vi "Update Data File to add Financials.vi"() -> ()   [LabVIEW 2020]
uses:
  WPC Player and Financial Stats.ctl
panel:
  in  "file path (use dialog)":path=path "G:/My Drive/WPC Stat Scrape/Data/WPC Stats.bin"
  out "error out":errorcluster
  out "WPC Player and Financial Stats":T1[][](array[typedef])=[[{"Player Name"="Andrew", "Date Updated"=timestamp(3695932800 s since 1904-01-01), "Tournament Stats"={"Hands Won"=674, "Hands Played"=2024, "Hands Dealt"=5109, "All-Ins"=149, "Entered"=36, "Winnings"=785.66, "Profit"=-679.15}, "Cash Stats"={"Hands Won"=1363, "Hands Played"=4015, "Hands Dealt"=9376, "All-Ins"=232, "Profit"=-195.0}}, {"Player Name"="Brian", "Date Updated"=timestamp(3695932800 s since 1904-01-01), "Tournament Stats"={"Hands Won"=936, "Hands Played"=2541, "Hands Dealt"=5628, "All-Ins"=306, "Entered"=47, "Winnings"=1307.11, "Profit"=-47.7}, "Cash Stats"={"Hands Won"=2327, "Hands Played"=6457, "Hands Dealt"=11257, "All-Ins"=405, "Profit"=1902.25}}, {"Player Name"="Daniel", "Date Updated"=timestamp(3695932800 s since 1904-01-01), "Tournament Stats"={"Hands Won"=94, "Hands Played"=308, "Hands Dealt"=723, "All-Ins"=23, "Entered"=6, "Winnings"=320.0, "Profit"=-20.0}, "Cash Stats"={"Hands Won"=0, "Hands Played"=0, "Hands Dealt"=0, "All-Ins"=0, "Profit"=0.0}}, {"Player Name"="David", "Date Updated"=timestamp(3695932800 s since 1904-01-01), "Tournament Stats"={"Hands Won"=898, "Hands Played"=2002, "Hands Dealt"=4936, "All-Ins"=188, "Entered"=37, "Winnings"=1934.16, "Profit"=574.16}, "Cash Stats"={"Hands Won"=0, "Hands Played"=0, "Hands Dealt"=0, "All-Ins"=0, "Profit"=0.0}}, {"Player Name"="Dennis", "Date Updated"=timestamp(3695932800 s since 1904-01-01), "Tournament Stats"={"Hands Won"=266, "Hands Played"=670, "Hands Dealt"=1843, "All-Ins"=55, "Entered"=13, "Winnings"=1351.83, "Profit"=617.02}, "Cash Stats"={"Hands Won"=34, "Hands Played"=114, "Hands Dealt"=216, "All-Ins"=11, "Profit"=-12.75}}, {"Player Name"="Doug", "Date Updated"=timestamp(3695932800 s since 1904-01-01), "Tournament Stats"={"Hands Won"=144, "Hands Played"=441, "Hands Dealt"=722, "All-Ins"=44, "Entered"=11, "Winnings"=225.0, "Profit"=-89.81}, "Cash Stats"={"Hands Won"=120, "Hands Played"=285, "Hands Dealt"=428, "All-Ins"=22, "Profit"=-39.5}}, {"Player Name"="Erik", "Date Updated"=timestamp(3695932800 s since 1904-01-01), "Tournament Stats"={"Hands Won"=180, "Hands Played"=626, "Hands Dealt"=1825, "All-Ins"=72, "Entered"=14, "Winnings"=200.66, "Profit"=-259.34}, "Cash Stats"={"Hands Won"=11, "Hands Played"=43, "Hands Dealt"=98, "All-Ins"=7, "Profit"=-34.75}}, {"Player Name"="Ethan", "Date Updated"=timestamp(3695932800 s since 1904-01-01), "Tournament Stats"={"Hands Won"=735, "Hands Played"=2022, "Hands Dealt"=5107, "All-Ins"=210, "Entered"=41, "Winnings"=1270.72, "Profit"=195.91}, "Cash Stats"={"Hands Won"=2067, "Hands Played"=5488, "Hands Dealt"=10831, "All-Ins"=624, "Profit"=1356.0}}, {"Player Name"="Ian", "Date Updated"=timestamp(3695932800 s since 1904-01-01), "Tournament Stats"={"Hands Won"=1572, "Hands Played"=4650, "Hands Dealt"=8870, "All-Ins"=332, "Entered"=69, "Winnings"=1957.52, "Profit"=-407.29}, "Cash Stats"={"Hands Won"=129, "Hands Played"=435, "Hands Dealt"=646, "All-Ins"=23, "Profit"=-112.0}}, {"Player Name"="Ira", "Date Updated"=timestamp(3695932800 s since 1904-01-01), "Tournament Stats"={"Hands Won"=1430, "Hands Played"=3509, "Hands Dealt"=8784, "All-Ins"=341, "Entered"=72, "Winnings"=2796.14, "Profit"=491.33}, "Cash Stats"={"Hands Won"=1, "Hands Played"=3, "Hands Dealt"=6, "All-Ins"=1, "Profit"=-20.0}}, {"Player Name"="Jason", "Date Updated"=timestamp(3695932800 s since 1904-01-01), "Tournament Stats"={"Hands Won"=137, "Hands Played"=440, "Hands Dealt"=846, "All-Ins"=37, "Entered"=10, "Winnings"=56.0, "Profit"=-324.0}, "Cash Stats"={"Hands Won"=87, "Hands Played"=305, "Hands Dealt"=448, "All-Ins"=19, "Profit"=-77.75}}, {"Player Name"="Jeff", "Date Updated"=timestamp(3695932800 s since 1904-01-01), "Tournament Stats"={"Hands Won"=445, "Hands Played"=1629, "Hands Dealt"=3147, "All-Ins"=145, "Entered"=39, "Winnings"=420.0, "Profit"=-584.81}, "Cash Stats"={"Hands Won"=0, "Hands Played"=0, "Hands Dealt"=0, "All-Ins"=0, "Profit"=0.0}}, {"Player Name"="Jeff-R", "Date Updated"=timestamp(3695932800 s since 1904-01-01), "Tournament Stats"={"Hands Won"=134, "Hands Played"=331, "Hands Dealt"=875, "All-Ins"=43, "Entered"=7, "Winnings"=256.66, "Profit"=-3.34}, "Cash Stats"={"Hands Won"=10, "Hands Played"=25, "Hands Dealt"=60, "All-Ins"=3, "Profit"=-40.0}}, {"Player Name"="Joe", "Date Updated"=timestamp(3695932800 s since 1904-01-01), "Tournament Stats"={"Hands Won"=7, "Hands Played"=25, "Hands Dealt"=96, "All-Ins"=4, "Entered"=1, "Winnings"=0.0, "Profit"=-60.0}, "Cash Stats"={"Hands Won"=40, "Hands Played"=136, "Hands Dealt"=192, "All-Ins"=13, "Profit"=-132.5}}, {"Player Name"="Joe-Hockman", "Date Updated"=timestamp(3695932800 s since 1904-01-01), "Tournament Stats"={"Hands Won"=0, "Hands Played"=0, "Hands Dealt"=0, "All-Ins"=0, "Entered"=0, "Winnings"=0.0, "Profit"=-40.0}, "Cash Stats"={"Hands Won"=0, "Hands Played"=0, "Hands Dealt"=0, "All-Ins"=0, "Profit"=0.0}}, {"Player Name"="Jonathan-H", "Date Updated"=timestamp(3695932800 s since 1904-01-01), "Tournament Stats"={"Hands Won"=1295, "Hands Played"=2760, "Hands Dealt"=8906, "All-Ins"=385, "Entered"=70, "Winnings"=3077.49, "Profit"=762.68}, "Cash Stats"={"Hands Won"=2243, "Hands Played"=5750, "Hands Dealt"=9974, "All-Ins"=451, "Profit"=1226.5}}, {"Player Name"="Jonathan-M", "Date Updated"=timestamp(3695932800 s since 1904-01-01), "Tournament Stats"={"Hands Won"=2012, "Hands Played"=4111, "Hands Dealt"=8961, "All-Ins"=623, "Entered"=72, "Winnings"=3723.66, "Profit"=1128.85}, "Cash Stats"={"Hands Won"=5567, "Hands Played"=10633, "Hands Dealt"=14708, "All-Ins"=1306, "Profit"=-4255.25}}, {"Player Name"="Mark", "Date Updated"=timestamp(3695932800 s since 1904-01-01), "Tournament Stats"={"Hands Won"=1072, "Hands Played"=2139, "Hands Dealt"=6063, "All-Ins"=291, "Entered"=43, "Winnings"=3075.83, "Profit"=1615.83}, "Cash Stats"={"Hands Won"=746, "Hands Played"=1778, "Hands Dealt"=3876, "All-Ins"=94, "Profit"=895.25}}, {"Player Name"="Marty", "Date Updated"=timestamp(3695932800 s since 1904-01-01), "Tournament Stats"={"Hands Won"=1333, "Hands Played"=3356, "Hands Dealt"=8693, "All-Ins"=359, "Entered"=63, "Winnings"=2027.99, "Profit"=197.99}, "Cash Stats"={"Hands Won"=177, "Hands Played"=535, "Hands Dealt"=1236, "All-Ins"=35, "Profit"=-120.25}}, {"Player Name"="Matt-H", "Date Updated"=timestamp(3695932800 s since 1904-01-01), "Tournament Stats"={"Hands Won"=54, "Hands Played"=147, "Hands Dealt"=285, "All-Ins"=9, "Entered"=4, "Winnings"=34.0, "Profit"=-66.0}, "Cash Stats"={"Hands Won"=0, "Hands Played"=0, "Hands Dealt"=0, "All-Ins"=0, "Profit"=0.0}}, {"Player Name"="Matt-R", "Date Updated"=timestamp(3695932800 s since 1904-01-01), "Tournament Stats"={"Hands Won"=1041, "Hands Played"=2491, "Hands Dealt"=7307, "All-Ins"=340, "Entered"=50, "Winnings"=1520.16, "Profit"=-274.65}, "Cash Stats"={"Hands Won"=264, "Hands Played"=640, "Hands Dealt"=1515, "All-Ins"=91, "Profit"=-121.0}}, {"Player Name"="MikeDolan", "Date Updated"=timestamp(3695932800 s since 1904-01-01), "Tournament Stats"={"Hands Won"=529, "Hands Played"=1505, "Hands Dealt"=3790, "All-Ins"=171, "Entered"=26, "Winnings"=1025.66, "Profit"=85.66}, "Cash Stats"={"Hands Won"=32, "Hands Played"=117, "Hands Dealt"=225, "All-Ins"=14, "Profit"=-66.0}}, {"Player Name"="Nate", "Date Updated"=timestamp(3695932800 s since 1904-01-01), "Tournament Stats"={"Hands Won"=184, "Hands Played"=494, "Hands Dealt"=1384, "All-Ins"=42, "Entered"=14, "Winnings"=234.0, "Profit"=-36.0}, "Cash Stats"={"Hands Won"=0, "Hands Played"=0, "Hands Dealt"=0, "All-Ins"=0, "Profit"=0.0}}, {"Player Name"="Oren", "Date Updated"=timestamp(3695932800 s since 1904-01-01), "Tournament Stats"={"Hands Won"=822, "Hands Played"=1902, "Hands Dealt"=5455, "All-Ins"=177, "Entered"=46, "Winnings"=1157.32, "Profit"=-497.49}, "Cash Stats"={"Hands Won"=19, "Hands Played"=76, "Hands Dealt"=168, "All-Ins"=10, "Profit"=-140.0}}, {"Player Name"="Tom", "Date Updated"=timestamp(3695932800 s since 1904-01-01), "Tournament Stats"={"Hands Won"=0, "Hands Played"=0, "Hands Dealt"=0, "All-Ins"=0, "Entered"=0, "Winnings"=0.0, "Profit"=-120.0}, "Cash Stats"={"Hands Won"=0, "Hands Played"=0, "Hands Dealt"=0, "All-Ins"=0, "Profit"=6.75}}], [{"Player Name"="Andrew", "Date Updated"=timestamp(3696278400 s since 1904-01-01), "Tournament Stats"={"Hands Won"=692, "Hands Played"=2072, "Hands Dealt"=5257, "All-Ins"=152, "Entered"=37, "Winnings"=785.66, "Profit"=-679.15}, "Cash Stats"={"Hands Won"=1438, "Hands Played"=4236, "Hands Dealt"=9848, "All-Ins"=241, "Profit"=-195.0}}, {"Player Name"="Brian", "Date Updated"=timestamp(3696278400 s since 1904-01-01), "Tournament Stats"={"Hands Won"=982, "Hands Played"=2638, "Hands Dealt"=5878, "All-Ins"=313, "Entered"=49, "Winnings"=1307.11, "Profit"=-47.7}, "Cash Stats"={"Hands Won"=2444, "Hands Played"=6799, "Hands Dealt"=11839, "All-Ins"=418, "Profit"=1902.25}}, {"Player Name"="Daniel", "Date Updated"=timestamp(3696278400 s since 1904-01-01), "Tournament Stats"={"Hands Won"=123, "Hands Played"=372, "Hands Dealt"=887, "All-Ins"=30, "Entered"=7, "Winnings"=320.0, "Profit"=-20.0}, "Cash Stats"={"Hands Won"=0, "Hands Played"=0, "Hands Dealt"=0, "All-Ins"=0, "Profit"=0.0}}, {"Player Name"="David", "Date Updated"=timestamp(3696278400 s since 1904-01-01), "Tournament Stats"={"Hands Won"=923, "Hands Played"=2058, "Hands Dealt"=5088, "All-Ins"=191, "Entered"=38, "Winnings"=1934.16, "Profit"=574.16}, "Cash Stats"={"Hands Won"=0, "Hands Played"=0, "Hands Dealt"=0, "All-Ins"=0, "Profit"=0.0}}, {"Player Name"="Dennis", "Date Updated"=timestamp(3696278400 s since 1904-01-01), "Tournament Stats"={"Hands Won"=291, "Hands Played"=736, "Hands Dealt"=2087, "All-Ins"=67, "Entered"=15, "Winnings"=1351.83, "Profit"=617.02}, "Cash Stats"={"Hands Won"=64, "Hands Played"=197, "Hands Dealt"=380, "All-Ins"=17, "Profit"=-12.75}}, {"Player Name"="Doug", "Date Updated"=timestamp(3696278400 s since 1904-01-01), "Tournament Stats"={"Hands Won"=144, "Hands Played"=441, "Hands Dealt"=722, "All-Ins"=44, "Entered"=11, "Winnings"=225.0, "Profit"=-89.81}, "Cash Stats"={"Hands Won"=120, "Hands Played"=285, "Hands Dealt"=428, "All-Ins"=22, "Profit"=-39.5}}, {"Player Name"="Erik", "Date Updated"=timestamp(3696278400 s since 1904-01-01), "Tournament Stats"={"Hands Won"=187, "Hands Played"=660, "Hands Dealt"=1934, "All-Ins"=74, "Entered"=15, "Winnings"=200.66, "Profit"=-259.34}, "Cash Stats"={"Hands Won"=11, "Hands Played"=43, "Hands Dealt"=98, "All-Ins"=7, "Profit"=-34.75}}, {"Player Name"="Ethan", "Date Updated"=timestamp(3696278400 s since 1904-01-01), "Tournament Stats"={"Hands Won"=781, "Hands Played"=2112, "Hands Dealt"=5289, "All-Ins"=214, "Entered"=42, "Winnings"=1270.72, "Profit"=195.91}, "Cash Stats"={"Hands Won"=2170, "Hands Played"=5765, "Hands Dealt"=11302, "All-Ins"=648, "Profit"=1356.0}}, {"Player Name"="Ian", "Date Updated"=timestamp(3696278400 s since 1904-01-01), "Tournament Stats"={"Hands Won"=1605, "Hands Played"=4769, "Hands Dealt"=9117, "All-Ins"=349, "Entered"=71, "Winnings"=1957.52, "Profit"=-407.29}, "Cash Stats"={"Hands Won"=131, "Hands Played"=450, "Hands Dealt"=675, "All-Ins"=24, "Profit"=-112.0}}, {"Player Name"="Ira", "Date Updated"=timestamp(3696278400 s since 1904-01-01), "Tournament Stats"={"Hands Won"=1453, "Hands Played"=3592, "Hands Dealt"=8981, "All-Ins"=350, "Entered"=74, "Winnings"=2796.14, "Profit"=491.33}, "Cash Stats"={"Hands Won"=1, "Hands Played"=3, "Hands Dealt"=6, "All-Ins"=1, "Profit"=-20.0}}, {"Player Name"="Jason", "Date Updated"=timestamp(3696278400 s since 1904-01-01), "Tournament Stats"={"Hands Won"=137, "Hands Played"=440, "Hands Dealt"=846, "All-Ins"=37, "Entered"=10, "Winnings"=56.0, "Profit"=-324.0}, "Cash Stats"={"Hands Won"=87, "Hands Played"=305, "Hands Dealt"=448, "All-Ins"=19, "Profit"=-77.75}}, {"Player Name"="Jeff", "Date Updated"=timestamp(3696278400 s since 1904-01-01), "Tournament Stats"={"Hands Won"=460, "Hands Played"=1685, "Hands Dealt"=3258, "All-Ins"=150, "Entered"=40, "Winnings"=420.0, "Profit"=-584.81}, "Cash Stats"={"Hands Won"=0, "Hands Played"=0, "Hands Dealt"=0, "All-Ins"=0, "Profit"=0.0}}, {"Player Name"="Jeff-R", "Date Updated"=timestamp(3696278400 s since 1904-01-01), "Tournament Stats"={"Hands Won"=134, "Hands Played"=331, "Hands Dealt"=875, "All-Ins"=43, "Entered"=7, "Winnings"=256.66, "Profit"=-3.34}, "Cash Stats"={"Hands Won"=10, "Hands Played"=25, "Hands Dealt"=60, "All-Ins"=3, "Profit"=-40.0}}, {"Player Name"="Joe", "Date Updated"=timestamp(3696278400 s since 1904-01-01), "Tournament Stats"={"Hands Won"=7, "Hands Played"=25, "Hands Dealt"=96, "All-Ins"=4, "Entered"=1, "Winnings"=0.0, "Profit"=-60.0}, "Cash Stats"={"Hands Won"=40, "Hands Played"=136, "Hands Dealt"=192, "All-Ins"=13, "Profit"=-132.5}}, {"Player Name"="Joe-Hockman", "Date Updated"=timestamp(3696278400 s since 1904-01-01), "Tournament Stats"={"Hands Won"=0, "Hands Played"=0, "Hands Dealt"=0, "All-Ins"=0, "Entered"=0, "Winnings"=0.0, "Profit"=-40.0}, "Cash Stats"={"Hands Won"=0, "Hands Played"=0, "Hands Dealt"=0, "All-Ins"=0, "Profit"=0.0}}, {"Player Name"="Jonathan-H", "Date Updated"=timestamp(3696278400 s since 1904-01-01), "Tournament Stats"={"Hands Won"=1355, "Hands Played"=2840, "Hands Dealt"=9179, "All-Ins"=393, "Entered"=72, "Winnings"=3077.49, "Profit"=762.68}, "Cash Stats"={"Hands Won"=2263, "Hands Played"=5817, "Hands Dealt"=10092, "All-Ins"=461, "Profit"=1226.5}}, {"Player Name"="Jonathan-M", "Date Updated"=timestamp(3696278400 s since 1904-01-01), "Tournament Stats"={"Hands Won"=2058, "Hands Played"=4217, "Hands Dealt"=9164, "All-Ins"=642, "Entered"=74, "Winnings"=3723.66, "Profit"=1128.85}, "Cash Stats"={"Hands Won"=5684, "Hands Played"=10939, "Hands Dealt"=15071, "All-Ins"=1333, "Profit"=-4255.25}}, {"Player Name"="Mark", "Date Updated"=timestamp(3696278400 s since 1904-01-01), "Tournament Stats"={"Hands Won"=1081, "Hands Played"=2168, "Hands Dealt"=6180, "All-Ins"=297, "Entered"=44, "Winnings"=3075.83, "Profit"=1615.83}, "Cash Stats"={"Hands Won"=836, "Hands Played"=1984, "Hands Dealt"=4426, "All-Ins"=100, "Profit"=895.25}}, {"Player Name"="Marty", "Date Updated"=timestamp(3696278400 s since 1904-01-01), "Tournament Stats"={"Hands Won"=1391, "Hands Played"=3485, "Hands Dealt"=9040, "All-Ins"=374, "Entered"=65, "Winnings"=2027.99, "Profit"=197.99}, "Cash Stats"={"Hands Won"=189, "Hands Played"=570, "Hands Dealt"=1351, "All-Ins"=38, "Profit"=-120.25}}, {"Player Name"="Matt-H", "Date Updated"=timestamp(3696278400 s since 1904-01-01), "Tournament Stats"={"Hands Won"=54, "Hands Played"=147, "Hands Dealt"=285, "All-Ins"=9, "Entered"=4, "Winnings"=34.0, "Profit"=-66.0}, "Cash Stats"={"Hands Won"=0, "Hands Played"=0, "Hands Dealt"=0, "All-Ins"=0, "Profit"=0.0}}, {"Player Name"="Matt-R", "Date Updated"=timestamp(3696278400 s since 1904-01-01), "Tournament Stats"={"Hands Won"=1056, "Hands Played"=2563, "Hands Dealt"=7489, "All-Ins"=347, "Entered"=52, "Winnings"=1520.16, "Profit"=-274.65}, "Cash Stats"={"Hands Won"=264, "Hands Played"=640, "Hands Dealt"=1515, "All-Ins"=91, "Profit"=-121.0}}, {"Player Name"="MikeDolan", "Date Updated"=timestamp(3696278400 s since 1904-01-01), "Tournament Stats"={"Hands Won"=555, "Hands Played"=1565, "Hands Dealt"=3960, "All-Ins"=178, "Entered"=27, "Winnings"=1025.66, "Profit"=85.66}, "Cash Stats"={"Hands Won"=32, "Hands Played"=117, "Hands Dealt"=225, "All-Ins"=14, "Profit"=-66.0}}, {"Player Name"="Nate", "Date Updated"=timestamp(3696278400 s since 1904-01-01), "Tournament Stats"={"Hands Won"=184, "Hands Played"=494, "Hands Dealt"=1384, "All-Ins"=42, "Entered"=14, "Winnings"=234.0, "Profit"=-36.0}, "Cash Stats"={"Hands Won"=0, "Hands Played"=0, "Hands Dealt"=0, "All-Ins"=0, "Profit"=0.0}}, {"Player Name"="Oren", "Date Updated"=timestamp(3696278400 s since 1904-01-01), "Tournament Stats"={"Hands Won"=850, "Hands Played"=1972, "Hands Dealt"=5639, "All-Ins"=182, "Entered"=48, "Winnings"=1157.32, "Profit"=-497.49}, "Cash Stats"={"Hands Won"=19, "Hands Played"=76, "Hands Dealt"=168, "All-Ins"=10, "Profit"=-140.0}}, {"Player Name"="Tom", "Date Updated"=timestamp(3696278400 s since 1904-01-01), "Tournament Stats"={"Hands Won"=0, "Hands Played"=0, "Hands Dealt"=0, "All-Ins"=0, "Entered"=0, "Winnings"=0.0, "Profit"=-120.0}, "Cash Stats"={"Hands Won"=0, "Hands Played"=0, "Hands Dealt"=0, "All-Ins"=0, "Profit"=6.75}}], [{"Player Name"="Andrew", "Date Updated"=timestamp(3696883200 s since 1904-01-01), "Tournament Stats"={"Hands Won"=703, "Hands Played"=2106, "Hands Dealt"=5350, "All-Ins"=156, "Entered"=38, "Winnings"=785.66, "Profit"=-679.15}, "Cash Stats"={"Hands Won"=1504, "Hands Played"=4457, "Hands Dealt"=10311, "All-Ins"=259, "Profit"=-195.0}}, {"Player Name"="Brian", "Date Updated"=timestamp(3696883200 s since 1904-01-01), "Tournament Stats"={"Hands Won"=989, "Hands Played"=2670, "Hands Dealt"=5940, "All-Ins"=317, "Entered"=50, "Winnings"=1307.11, "Profit"=-47.7}, "Cash Stats"={"Hands Won"=2519, "Hands Played"=7033, "Hands Dealt"=12257, "All-Ins"=421, "Profit"=1902.25}}, {"Player Name"="Daniel", "Date Updated"=timestamp(3696883200 s since 1904-01-01), "Tournament Stats"={"Hands Won"=123, "Hands Played"=372, "Hands Dealt"=887, "All-Ins"=30, "Entered"=7, "Winnings"=320.0, "Profit"=-20.0}, "Cash Stats"={"Hands Won"=0, "Hands Played"=0, "Hands Dealt"=0, "All-Ins"=0, "Profit"=0.0}}, {"Player Name"="David", "Date Updated"=timestamp(3696883200 s since 1904-01-01), "Tournament Stats"={"Hands Won"=930, "Hands Played"=2085, "Hands Dealt"=5181, "All-Ins"=193, "Entered"=39, "Winnings"=1934.16, "Profit"=574.16}, "Cash Stats"={"Hands Won"=0, "Hands Played"=0, "Hands Dealt"=0, "All-Ins"=0, "Profit"=0.0}}, {"Player Name"="Dennis", "Date Updated"=timestamp(3696883200 s since 1904-01-01), "Tournament Stats"={"Hands Won"=319, "Hands Played"=819, "Hands Dealt"=2303, "All-Ins"=72, "Entered"=17, "Winnings"=1351.83, "Profit"=617.02}, "Cash Stats"={"Hands Won"=70, "Hands Played"=213, "Hands Dealt"=407, "All-Ins"=21, "Profit"=-12.75}}, {"Player Name"="Doug", "Date Updated"=timestamp(3696883200 s since 1904-01-01), "Tournament Stats"={"Hands Won"=157, "Hands Played"=475, "Hands Dealt"=808, "All-Ins"=48, "Entered"=12, "Winnings"=225.0, "Profit"=-89.81}, "Cash Stats"={"Hands Won"=120, "Hands Played"=285, "Hands Dealt"=428, "All-Ins"=22, "Profit"=-39.5}}, {"Player Name"="Erik", "Date Updated"=timestamp(3696883200 s since 1904-01-01), "Tournament Stats"={"Hands Won"=187, "Hands Played"=660, "Hands Dealt"=1934, "All-Ins"=74, "Entered"=15, "Winnings"=200.66, "Profit"=-259.34}, "Cash Stats"={"Hands Won"=11, "Hands Played"=43, "Hands Dealt"=98, "All-Ins"=7, "Profit"=-34.75}}, {"Player Name"="Ethan", "Date Updated"=timestamp(3696883200 s since 1904-01-01), "Tournament Stats"={"Hands Won"=847, "Hands Played"=2260, "Hands Dealt"=5600, "All-Ins"=229, "Entered"=44, "Winnings"=1270.72, "Profit"=195.91}, "Cash Stats"={"Hands Won"=2319, "Hands Played"=6069, "Hands Dealt"=11823, "All-Ins"=660, "Profit"=1356.0}}, {"Player Name"="Ian", "Date Updated"=timestamp(3696883200 s since 1904-01-01), "Tournament Stats"={"Hands Won"=1650, "Hands Played"=4899, "Hands Dealt"=9371, "All-Ins"=357, "Entered"=73, "Winnings"=1957.52, "Profit"=-407.29}, "Cash Stats"={"Hands Won"=177, "Hands Played"=584, "Hands Dealt"=866, "All-Ins"=25, "Profit"=-112.0}}, {"Player Name"="Ira", "Date Updated"=timestamp(3696883200 s since 1904-01-01), "Tournament Stats"={"Hands Won"=1477, "Hands Played"=3674, "Hands Dealt"=9138, "All-Ins"=360, "Entered"=76, "Winnings"=2796.14, "Profit"=491.33}, "Cash Stats"={"Hands Won"=1, "Hands Played"=3, "Hands Dealt"=6, "All-Ins"=1, "Profit"=-20.0}}, {"Player Name"="Jason", "Date Updated"=timestamp(3696883200 s since 1904-01-01), "Tournament Stats"={"Hands Won"=137, "Hands Played"=440, "Hands Dealt"=846, "All-Ins"=37, "Entered"=10, "Winnings"=56.0, "Profit"=-324.0}, "Cash Stats"={"Hands Won"=87, "Hands Played"=305, "Hands Dealt"=448, "All-Ins"=19, "Profit"=-77.75}}, {"Player Name"="Jeff", "Date Updated"=timestamp(3696883200 s since 1904-01-01), "Tournament Stats"={"Hands Won"=477, "Hands Played"=1738, "Hands Dealt"=3360, "All-Ins"=155, "Entered"=42, "Winnings"=420.0, "Profit"=-584.81}, "Cash Stats"={"Hands Won"=0, "Hands Played"=0, "Hands Dealt"=0, "All-Ins"=0, "Profit"=0.0}}, {"Player Name"="Jeff-R", "Date Updated"=timestamp(3696883200 s since 1904-01-01), "Tournament Stats"={"Hands Won"=139, "Hands Played"=345, "Hands Dealt"=913, "All-Ins"=45, "Entered"=8, "Winnings"=256.66, "Profit"=-3.34}, "Cash Stats"={"Hands Won"=10, "Hands Played"=25, "Hands Dealt"=60, "All-Ins"=3, "Profit"=-40.0}}, {"Player Name"="Joe", "Date Updated"=timestamp(3696883200 s since 1904-01-01), "Tournament Stats"={"Hands Won"=7, "Hands Played"=25, "Hands Dealt"=96, "All-Ins"=4, "Entered"=1, "Winnings"=0.0, "Profit"=-60.0}, "Cash Stats"={"Hands Won"=40, "Hands Played"=136, "Hands Dealt"=192, "All-Ins"=13, "Profit"=-132.5}}, {"Player Name"="Joe-Hockman", "Date Updated"=timestamp(3696883200 s since 1904-01-01), "Tournament Stats"={"Hands Won"=0, "Hands Played"=0, "Hands Dealt"=0, "All-Ins"=0, "Entered"=0, "Winnings"=0.0, "Profit"=-40.0}, "Cash Stats"={"Hands Won"=0, "Hands Played"=0, "Hands Dealt"=0, "All-Ins"=0, "Profit"=0.0}}, {"Player Name"="Jonathan-H", "Date Updated"=timestamp(3696883200 s since 1904-01-01), "Tournament Stats"={"Hands Won"=1402, "Hands Played"=2937, "Hands Dealt"=9447, "All-Ins"=402, "Entered"=74, "Winnings"=3077.49, "Profit"=762.68}, "Cash Stats"={"Hands Won"=2319, "Hands Played"=5993, "Hands Dealt"=10405, "All-Ins"=481, "Profit"=1226.5}}, {"Player Name"="Jonathan-M", "Date Updated"=timestamp(3696883200 s since 1904-01-01), "Tournament Stats"={"Hands Won"=2102, "Hands Played"=4317, "Hands Dealt"=9385, "All-Ins"=652, "Entered"=76, "Winnings"=3723.66, "Profit"=1128.85}, "Cash Stats"={"Hands Won"=5831, "Hands Played"=11248, "Hands Dealt"=15514, "All-Ins"=1377, "Profit"=-4255.25}}, {"Player Name"="Mark", "Date Updated"=timestamp(3696883200 s since 1904-01-01), "Tournament Stats"={"Hands Won"=1129, "Hands Played"=2254, "Hands Dealt"=6431, "All-Ins"=301, "Entered"=46, "Winnings"=3075.83, "Profit"=1615.83}, "Cash Stats"={"Hands Won"=879, "Hands Played"=2069, "Hands Dealt"=4633, "All-Ins"=103, "Profit"=895.25}}, {"Player Name"="Marty", "Date Updated"=timestamp(3696883200 s since 1904-01-01), "Tournament Stats"={"Hands Won"=1438, "Hands Played"=3592, "Hands Dealt"=9336, "All-Ins"=388, "Entered"=67, "Winnings"=2027.99, "Profit"=197.99}, "Cash Stats"={"Hands Won"=220, "Hands Played"=667, "Hands Dealt"=1529, "All-Ins"=40, "Profit"=-120.25}}, {"Player Name"="Matt-H", "Date Updated"=timestamp(3696883200 s since 1904-01-01), "Tournament Stats"={"Hands Won"=54, "Hands Played"=147, "Hands Dealt"=285, "All-Ins"=9, "Entered"=4, "Winnings"=34.0, "Profit"=-66.0}, "Cash Stats"={"Hands Won"=0, "Hands Played"=0, "Hands Dealt"=0, "All-Ins"=0, "Profit"=0.0}}, {"Player Name"="Matt-R", "Date Updated"=timestamp(3696883200 s since 1904-01-01), "Tournament Stats"={"Hands Won"=1089, "Hands Played"=2669, "Hands Dealt"=7742, "All-Ins"=362, "Entered"=54, "Winnings"=1520.16, "Profit"=-274.65}, "Cash Stats"={"Hands Won"=268, "Hands Played"=653, "Hands Dealt"=1540, "All-Ins"=96, "Profit"=-121.0}}, {"Player Name"="MikeDolan", "Date Updated"=timestamp(3696883200 s since 1904-01-01), "Tournament Stats"={"Hands Won"=571, "Hands Played"=1608, "Hands Dealt"=4082, "All-Ins"=181, "Entered"=28, "Winnings"=1025.66, "Profit"=85.66}, "Cash Stats"={"Hands Won"=32, "Hands Played"=117, "Hands Dealt"=225, "All-Ins"=14, "Profit"=-66.0}}, {"Player Name"="Nate", "Date Updated"=timestamp(3696883200 s since 1904-01-01), "Tournament Stats"={"Hands Won"=184, "Hands Played"=494, "Hands Dealt"=1384, "All-Ins"=42, "Entered"=14, "Winnings"=234.0, "Profit"=-36.0}, "Cash Stats"={"Hands Won"=0, "Hands Played"=0, "Hands Dealt"=0, "All-Ins"=0, "Profit"=0.0}}, {"Player Name"="Oren", "Date Updated"=timestamp(3696883200 s since 1904-01-01), "Tournament Stats"={"Hands Won"=878, "Hands Played"=2040, "Hands Dealt"=5788, "All-Ins"=188, "Entered"=49, "Winnings"=1157.32, "Profit"=-497.49}, "Cash Stats"={"Hands Won"=19, "Hands Played"=76, "Hands Dealt"=168, "All-Ins"=10, "Profit"=-140.0}}, {"Player Name"="Tom", "Date Updated"=timestamp(3696883200 s since 1904-01-01), "Tournament Stats"={"Hands Won"=0, "Hands Played"=0, "Hands Dealt"=0, "All-Ins"=0, "Entered"=0, "Winnings"=0.0, "Profit"=-120.0}, "Cash Stats"={"Hands Won"=0, "Hands Played"=0, "Hands Dealt"=0, "All-Ins"=0, "Profit"=6.75}}], [{"Player Name"="Andrew", "Date Updated"=timestamp(3697488000 s since 1904-01-01), "Tournament Stats"={"Hands Won"=731, "Hands Played"=2173, "Hands Dealt"=5555, "All-Ins"=165, "Entered"=39, "Winnings"=785.66, "Profit"=-679.15}, "Cash Stats"={"Hands Won"=1573, "Hands Played"=4704, "Hands Dealt"=10887, "All-Ins"=278, "Profit"=-195.0}}, {"Player Name"="Brian", "Date Updated"=timestamp(3697488000 s since 1904-01-01), "Tournament Stats"={"Hands Won"=1016, "Hands Played"=2750, "Hands Dealt"=6150, "All-Ins"=324, "Entered"=52, "Winnings"=1307.11, "Profit"=-47.7}, "Cash Stats"={"Hands Won"=2612, "Hands Played"=7326, "Hands Dealt"=12771, "All-Ins"=429, "Profit"=1902.25}}, {"Player Name"="Daniel", "Date Updated"=timestamp(3697488000 s since 1904-01-01), "Tournament Stats"={"Hands Won"=164, "Hands Played"=448, "Hands Dealt"=1126, "All-Ins"=35, "Entered"=8, "Winnings"=320.0, "Profit"=-20.0}, "Cash Stats"={"Hands Won"=0, "Hands Played"=0, "Hands Dealt"=0, "All-Ins"=0, "Profit"=0.0}}, {"Player Name"="David", "Date Updated"=timestamp(3697488000 s since 1904-01-01), "Tournament Stats"={"Hands Won"=973, "Hands Played"=2166, "Hands Dealt"=5422, "All-Ins"=201, "Entered"=40, "Winnings"=1934.16, "Profit"=574.16}, "Cash Stats"={"Hands Won"=0, "Hands Played"=0, "Hands Dealt"=0, "All-Ins"=0, "Profit"=0.0}}, {"Player Name"="Dennis", "Date Updated"=timestamp(3697488000 s since 1904-01-01), "Tournament Stats"={"Hands Won"=325, "Hands Played"=848, "Hands Dealt"=2428, "All-Ins"=77, "Entered"=18, "Winnings"=1351.83, "Profit"=617.02}, "Cash Stats"={"Hands Won"=77, "Hands Played"=234, "Hands Dealt"=452, "All-Ins"=25, "Profit"=-12.75}}, {"Player Name"="Doug", "Date Updated"=timestamp(3697488000 s since 1904-01-01), "Tournament Stats"={"Hands Won"=173, "Hands Played"=514, "Hands Dealt"=936, "All-Ins"=57, "Entered"=13, "Winnings"=225.0, "Profit"=-89.81}, "Cash Stats"={"Hands Won"=120, "Hands Played"=285, "Hands Dealt"=428, "All-Ins"=22, "Profit"=-39.5}}, {"Player Name"="Erik", "Date Updated"=timestamp(3697488000 s since 1904-01-01), "Tournament Stats"={"Hands Won"=195, "Hands Played"=696, "Hands Dealt"=2040, "All-Ins"=80, "Entered"=16, "Winnings"=200.66, "Profit"=-259.34}, "Cash Stats"={"Hands Won"=11, "Hands Played"=43, "Hands Dealt"=98, "All-Ins"=7, "Profit"=-34.75}}, {"Player Name"="Ethan", "Date Updated"=timestamp(3697488000 s since 1904-01-01), "Tournament Stats"={"Hands Won"=886, "Hands Played"=2371, "Hands Dealt"=5818, "All-Ins"=240, "Entered"=46, "Winnings"=1270.72, "Profit"=195.91}, "Cash Stats"={"Hands Won"=2563, "Hands Played"=6624, "Hands Dealt"=12741, "All-Ins"=735, "Profit"=1356.0}}, {"Player Name"="Ian", "Date Updated"=timestamp(3697488000 s since 1904-01-01), "Tournament Stats"={"Hands Won"=1679, "Hands Played"=5012, "Hands Dealt"=9609, "All-Ins"=369, "Entered"=75, "Winnings"=1957.52, "Profit"=-407.29}, "Cash Stats"={"Hands Won"=205, "Hands Played"=719, "Hands Dealt"=1100, "All-Ins"=26, "Profit"=-112.0}}, {"Player Name"="Ira", "Date Updated"=timestamp(3697488000 s since 1904-01-01), "Tournament Stats"={"Hands Won"=1530, "Hands Played"=3801, "Hands Dealt"=9427, "All-Ins"=372, "Entered"=78, "Winnings"=2796.14, "Profit"=491.33}, "Cash Stats"={"Hands Won"=1, "Hands Played"=3, "Hands Dealt"=6, "All-Ins"=1, "Profit"=-20.0}}, {"Player Name"="Jason", "Date Updated"=timestamp(3697488000 s since 1904-01-01), "Tournament Stats"={"Hands Won"=137, "Hands Played"=440, "Hands Dealt"=846, "All-Ins"=37, "Entered"=10, "Winnings"=56.0, "Profit"=-324.0}, "Cash Stats"={"Hands Won"=87, "Hands Played"=305, "Hands Dealt"=448, "All-Ins"=19, "Profit"=-77.75}}, {"Player Name"="Jeff", "Date Updated"=timestamp(3697488000 s since 1904-01-01), "Tournament Stats"={"Hands Won"=479, "Hands Played"=1762, "Hands Dealt"=3416, "All-Ins"=161, "Entered"=44, "Winnings"=420.0, "Profit"=-584.81}, "Cash Stats"={"Hands Won"=0, "Hands Played"=0, "Hands Dealt"=0, "All-Ins"=0, "Profit"=0.0}}, {"Player Name"="Jeff-R", "Date Updated"=timestamp(3697488000 s since 1904-01-01), "Tournament Stats"={"Hands Won"=163, "Hands Played"=398, "Hands Dealt"=1069, "All-Ins"=48, "Entered"=9, "Winnings"=256.66, "Profit"=-3.34}, "Cash Stats"={"Hands Won"=10, "Hands Played"=25, "Hands Dealt"=60, "All-Ins"=3, "Profit"=-40.0}}, {"Player Name"="Joe", "Date Updated"=timestamp(3697488000 s since 1904-01-01), "Tournament Stats"={"Hands Won"=7, "Hands Played"=25, "Hands Dealt"=96, "All-Ins"=4, "Entered"=1, "Winnings"=0.0, "Profit"=-60.0}, "Cash Stats"={"Hands Won"=40, "Hands Played"=136, "Hands Dealt"=192, "All-Ins"=13, "Profit"=-132.5}}, {"Player Name"="Joe-Hockman", "Date Updated"=timestamp(3697488000 s since 1904-01-01), "Tournament Stats"={"Hands Won"=0, "Hands Played"=0, "Hands Dealt"=0, "All-Ins"=0, "Entered"=0, "Winnings"=0.0, "Profit"=-40.0}, "Cash Stats"={"Hands Won"=0, "Hands Played"=0, "Hands Dealt"=0, "All-Ins"=0, "Profit"=0.0}}, {"Player Name"="Jonathan-H", "Date Updated"=timestamp(3697488000 s since 1904-01-01), "Tournament Stats"={"Hands Won"=1423, "Hands Played"=2997, "Hands Dealt"=9669, "All-Ins"=412, "Entered"=76, "Winnings"=3077.49, "Profit"=762.68}, "Cash Stats"={"Hands Won"=2418, "Hands Played"=6224, "Hands Dealt"=10925, "All-Ins"=489, "Profit"=1226.5}}, {"Player Name"="Jonathan-M", "Date Updated"=timestamp(3697488000 s since 1904-01-01), "Tournament Stats"={"Hands Won"=2172, "Hands Played"=4448, "Hands Dealt"=9705, "All-Ins"=666, "Entered"=78, "Winnings"=3723.66, "Profit"=1128.85}, "Cash Stats"={"Hands Won"=6177, "Hands Played"=11852, "Hands Dealt"=16386, "All-Ins"=1413, "Profit"=-4255.25}}, {"Player Name"="Mark", "Date Updated"=timestamp(3697488000 s since 1904-01-01), "Tournament Stats"={"Hands Won"=1174, "Hands Played"=2337, "Hands Dealt"=6703, "All-Ins"=309, "Entered"=48, "Winnings"=3075.83, "Profit"=1615.83}, "Cash Stats"={"Hands Won"=925, "Hands Played"=2185, "Hands Dealt"=4945, "All-Ins"=105, "Profit"=895.25}}, {"Player Name"="Marty", "Date Updated"=timestamp(3697488000 s since 1904-01-01), "Tournament Stats"={"Hands Won"=1480, "Hands Played"=3689, "Hands Dealt"=9630, "All-Ins"=404, "Entered"=69, "Winnings"=2027.99, "Profit"=197.99}, "Cash Stats"={"Hands Won"=238, "Hands Played"=704, "Hands Dealt"=1620, "All-Ins"=40, "Profit"=-120.25}}, {"Player Name"="Matt-H", "Date Updated"=timestamp(3697488000 s since 1904-01-01), "Tournament Stats"={"Hands Won"=54, "Hands Played"=147, "Hands Dealt"=285, "All-Ins"=9, "Entered"=4, "Winnings"=34.0, "Profit"=-66.0}, "Cash Stats"={"Hands Won"=0, "Hands Played"=0, "Hands Dealt"=0, "All-Ins"=0, "Profit"=0.0}}, {"Player Name"="Matt-R", "Date Updated"=timestamp(3697488000 s since 1904-01-01), "Tournament Stats"={"Hands Won"=1133, "Hands Played"=2784, "Hands Dealt"=8087, "All-Ins"=382, "Entered"=56, "Winnings"=1520.16, "Profit"=-274.65}, "Cash Stats"={"Hands Won"=273, "Hands Played"=667, "Hands Dealt"=1571, "All-Ins"=97, "Profit"=-121.0}}, {"Player Name"="MikeDolan", "Date Updated"=timestamp(3697488000 s since 1904-01-01), "Tournament Stats"={"Hands Won"=584, "Hands Played"=1648, "Hands Dealt"=4197, "All-Ins"=187, "Entered"=29, "Winnings"=1025.66, "Profit"=85.66}, "Cash Stats"={"Hands Won"=32, "Hands Played"=117, "Hands Dealt"=225, "All-Ins"=14, "Profit"=-66.0}}, {"Player Name"="Nate", "Date Updated"=timestamp(3697488000 s since 1904-01-01), "Tournament Stats"={"Hands Won"=184, "Hands Played"=494, "Hands Dealt"=1384, "All-Ins"=42, "Entered"=14, "Winnings"=234.0, "Profit"=-36.0}, "Cash Stats"={"Hands Won"=0, "Hands Played"=0, "Hands Dealt"=0, "All-Ins"=0, "Profit"=0.0}}, {"Player Name"="Oren", "Date Updated"=timestamp(3697488000 s since 1904-01-01), "Tournament Stats"={"Hands Won"=889, "Hands Played"=2082, "Hands Dealt"=5911, "All-Ins"=193, "Entered"=51, "Winnings"=1157.32, "Profit"=-497.49}, "Cash Stats"={"Hands Won"=19, "Hands Played"=76, "Hands Dealt"=168, "All-Ins"=10, "Profit"=-140.0}}, {"Player Name"="Tom", "Date Updated"=timestamp(3697488000 s since 1904-01-01), "Tournament Stats"={"Hands Won"=0, "Hands Played"=0, "Hands Dealt"=0, "All-Ins"=0, "Entered"=0, "Winnings"=0.0, "Profit"=-120.0}, "Cash Stats"={"Hands Won"=0, "Hands Played"=0, "Hands Dealt"=0, "All-Ins"=0, "Profit"=6.75}}], [{"Player Name"="Andrew", "Date Updated"=timestamp(3698092800 s since 1904-01-01), "Tournament Stats"={"Hands Won"=745, "Hands Played"=2228, "Hands Dealt"=5686, "All-Ins"=169, "Entered"=40, "Winnings"=785.66, "Profit"=-679.15}, "Cash Stats"={"Hands Won"=1691, "Hands Played"=5036, "Hands Dealt"=11645, "All-Ins"=300, "Profit"=-195.0}}, {"Player Name"="Brian", "Date Updated"=timestamp(3698092800 s since 1904-01-01), "Tournament Stats"={"Hands Won"=1049, "Hands Played"=2826, "Hands Dealt"=6323, "All-Ins"=331, "Entered"=53, "Winnings"=1307.11, "Profit"=-47.7}, "Cash Stats"={"Hands Won"=2712, "Hands Played"=7619, "Hands Dealt"=13310, "All-Ins"=444, "Profit"=1902.25}}, {"Player Name"="Daniel", "Date Updated"=timestamp(3698092800 s since 1904-01-01), "Tournament Stats"={"Hands Won"=173, "Hands Played"=476, "Hands Dealt"=1223, "All-Ins"=38, "Entered"=9, "Winnings"=320.0, "Profit"=-20.0}, "Cash Stats"={"Hands Won"=0, "Hands Played"=0, "Hands Dealt"=0, "All-Ins"=0, "Profit"=0.0}}, {"Player Name"="David", "Date Updated"=timestamp(3698092800 s since 1904-01-01), "Tournament Stats"={"Hands Won"=989, "Hands Played"=2209, "Hands Dealt"=5546, "All-Ins"=206, "Entered"=41, "Winnings"=1934.16, "Profit"=574.16}, "Cash Stats"={"Hands Won"=0, "Hands Played"=0, "Hands Dealt"=0, "All-Ins"=0, "Profit"=0.0}}, {"Player Name"="Dennis", "Date Updated"=timestamp(3698092800 s since 1904-01-01), "Tournament Stats"={"Hands Won"=390, "Hands Played"=991, "Hands Dealt"=2790, "All-Ins"=93, "Entered"=20, "Winnings"=1351.83, "Profit"=617.02}, "Cash Stats"={"Hands Won"=79, "Hands Played"=242, "Hands Dealt"=466, "All-Ins"=26, "Profit"=-12.75}}, {"Player Name"="Doug", "Date Updated"=timestamp(3698092800 s since 1904-01-01), "Tournament Stats"={"Hands Won"=191, "Hands Played"=550, "Hands Dealt"=1035, "All-Ins"=61, "Entered"=14, "Winnings"=225.0, "Profit"=-89.81}, "Cash Stats"={"Hands Won"=120, "Hands Played"=285, "Hands Dealt"=428, "All-Ins"=22, "Profit"=-39.5}}, {"Player Name"="Erik", "Date Updated"=timestamp(3698092800 s since 1904-01-01), "Tournament Stats"={"Hands Won"=195, "Hands Played"=696, "Hands Dealt"=2040, "All-Ins"=80, "Entered"=16, "Winnings"=200.66, "Profit"=-259.34}, "Cash Stats"={"Hands Won"=11, "Hands Played"=43, "Hands Dealt"=98, "All-Ins"=7, "Profit"=-34.75}}, {"Player Name"="Ethan", "Date Updated"=timestamp(3698092800 s since 1904-01-01), "Tournament Stats"={"Hands Won"=923, "Hands Played"=2482, "Hands Dealt"=6064, "All-Ins"=247, "Entered"=48, "Winnings"=1270.72, "Profit"=195.91}, "Cash Stats"={"Hands Won"=2681, "Hands Played"=6927, "Hands Dealt"=13273, "All-Ins"=760, "Profit"=1356.0}}, {"Player Name"="Ian", "Date Updated"=timestamp(3698092800 s since 1904-01-01), "Tournament Stats"={"Hands Won"=1727, "Hands Played"=5121, "Hands Dealt"=9854, "All-Ins"=377, "Entered"=77, "Winnings"=1957.52, "Profit"=-407.29}, "Cash Stats"={"Hands Won"=256, "Hands Played"=856, "Hands Dealt"=1326, "All-Ins"=27, "Profit"=-112.0}}, {"Player Name"="Ira", "Date Updated"=timestamp(3698092800 s since 1904-01-01), "Tournament Stats"={"Hands Won"=1563, "Hands Played"=3891, "Hands Dealt"=9600, "All-Ins"=380, "Entered"=80, "Winnings"=2796.14, "Profit"=491.33}, "Cash Stats"={"Hands Won"=1, "Hands Played"=3, "Hands Dealt"=6, "All-Ins"=1, "Profit"=-20.0}}, {"Player Name"="Jason", "Date Updated"=timestamp(3698092800 s since 1904-01-01), "Tournament Stats"={"Hands Won"=137, "Hands Played"=440, "Hands Dealt"=846, "All-Ins"=37, "Entered"=10, "Winnings"=56.0, "Profit"=-324.0}, "Cash Stats"={"Hands Won"=87, "Hands Played"=305, "Hands Dealt"=448, "All-Ins"=19, "Profit"=-77.75}}, {"Player Name"="Jeff", "Date Updated"=timestamp(3698092800 s since 1904-01-01), "Tournament Stats"={"Hands Won"=480, "Hands Played"=1783, "Hands Dealt"=3448, "All-Ins"=162, "Entered"=45, "Winnings"=420.0, "Profit"=-584.81}, "Cash Stats"={"Hands Won"=0, "Hands Played"=0, "Hands Dealt"=0, "All-Ins"=0, "Profit"=0.0}}, {"Player Name"="Jeff-R", "Date Updated"=timestamp(3698092800 s since 1904-01-01), "Tournament Stats"={"Hands Won"=163, "Hands Played"=398, "Hands Dealt"=1069, "All-Ins"=48, "Entered"=9, "Winnings"=256.66, "Profit"=-3.34}, "Cash Stats"={"Hands Won"=10, "Hands Played"=25, "Hands Dealt"=60, "All-Ins"=3, "Profit"=-40.0}}, {"Player Name"="Joe", "Date Updated"=timestamp(3698092800 s since 1904-01-01), "Tournament Stats"={"Hands Won"=7, "Hands Played"=25, "Hands Dealt"=96, "All-Ins"=4, "Entered"=1, "Winnings"=0.0, "Profit"=-60.0}, "Cash Stats"={"Hands Won"=40, "Hands Played"=136, "Hands Dealt"=192, "All-Ins"=13, "Profit"=-132.5}}, {"Player Name"="Joe-Hockman", "Date Updated"=timestamp(3698092800 s since 1904-01-01), "Tournament Stats"={"Hands Won"=3, "Hands Played"=26, "Hands Dealt"=56, "All-Ins"=2, "Entered"=1, "Winnings"=0.0, "Profit"=-40.0}, "Cash Stats"={"Hands Won"=0, "Hands Played"=0, "Hands Dealt"=0, "All-Ins"=0, "Profit"=0.0}}, {"Player Name"="Jonathan-H", "Date Updated"=timestamp(3698092800 s since 1904-01-01), "Tournament Stats"={"Hands Won"=1456, "Hands Played"=3067, "Hands Dealt"=9895, "All-Ins"=424, "Entered"=78, "Winnings"=3077.49, "Profit"=762.68}, "Cash Stats"={"Hands Won"=2527, "Hands Played"=6487, "Hands Dealt"=11380, "All-Ins"=505, "Profit"=1226.5}}, {"Player Name"="Jonathan-M", "Date Updated"=timestamp(3698092800 s since 1904-01-01), "Tournament Stats"={"Hands Won"=2303, "Hands Played"=4639, "Hands Dealt"=10158, "All-Ins"=695, "Entered"=80, "Winnings"=3723.66, "Profit"=1128.85}, "Cash Stats"={"Hands Won"=6370, "Hands Played"=12258, "Hands Dealt"=16919, "All-Ins"=1450, "Profit"=-4255.25}}, {"Player Name"="Mark", "Date Updated"=timestamp(3698092800 s since 1904-01-01), "Tournament Stats"={"Hands Won"=1220, "Hands Played"=2434, "Hands Dealt"=7003, "All-Ins"=324, "Entered"=50, "Winnings"=3075.83, "Profit"=1615.83}, "Cash Stats"={"Hands Won"=984, "Hands Played"=2323, "Hands Dealt"=5269, "All-Ins"=110, "Profit"=895.25}}, {"Player Name"="Marty", "Date Updated"=timestamp(3698092800 s since 1904-01-01), "Tournament Stats"={"Hands Won"=1533, "Hands Played"=3804, "Hands Dealt"=9931, "All-Ins"=415, "Entered"=71, "Winnings"=2027.99, "Profit"=197.99}, "Cash Stats"={"Hands Won"=242, "Hands Played"=729, "Hands Dealt"=1673, "All-Ins"=41, "Profit"=-120.25}}, {"Player Name"="Matt-H", "Date Updated"=timestamp(3698092800 s since 1904-01-01), "Tournament Stats"={"Hands Won"=54, "Hands Played"=147, "Hands Dealt"=285, "All-Ins"=9, "Entered"=4, "Winnings"=34.0, "Profit"=-66.0}, "Cash Stats"={"Hands Won"=0, "Hands Played"=0, "Hands Dealt"=0, "All-Ins"=0, "Profit"=0.0}}, {"Player Name"="Matt-R", "Date Updated"=timestamp(3698092800 s since 1904-01-01), "Tournament Stats"={"Hands Won"=1162, "Hands Played"=2870, "Hands Dealt"=8286, "All-Ins"=394, "Entered"=58, "Winnings"=1520.16, "Profit"=-274.65}, "Cash Stats"={"Hands Won"=288, "Hands Played"=709, "Hands Dealt"=1660, "All-Ins"=104, "Profit"=-121.0}}, {"Player Name"="MikeDolan", "Date Updated"=timestamp(3698092800 s since 1904-01-01), "Tournament Stats"={"Hands Won"=598, "Hands Played"=1696, "Hands Dealt"=4337, "All-Ins"=198, "Entered"=30, "Winnings"=1025.66, "Profit"=85.66}, "Cash Stats"={"Hands Won"=32, "Hands Played"=117, "Hands Dealt"=225, "All-Ins"=14, "Profit"=-66.0}}, {"Player Name"="Nate", "Date Updated"=timestamp(3698092800 s since 1904-01-01), "Tournament Stats"={"Hands Won"=184, "Hands Played"=494, "Hands Dealt"=1384, "All-Ins"=42, "Entered"=14, "Winnings"=234.0, "Profit"=-36.0}, "Cash Stats"={"Hands Won"=0, "Hands Played"=0, "Hands Dealt"=0, "All-Ins"=0, "Profit"=0.0}}, {"Player Name"="Oren", "Date Updated"=timestamp(3698092800 s since 1904-01-01), "Tournament Stats"={"Hands Won"=919, "Hands Played"=2146, "Hands Dealt"=6083, "All-Ins"=197, "Entered"=52, "Winnings"=1157.32, "Profit"=-497.49}, "Cash Stats"={"Hands Won"=19, "Hands Played"=76, "Hands Dealt"=168, "All-Ins"=10, "Profit"=-140.0}}, {"Player Name"="Tom", "Date Updated"=timestamp(3698092800 s since 1904-01-01), "Tournament Stats"={"Hands Won"=15, "Hands Played"=39, "Hands Dealt"=107, "All-Ins"=3, "Entered"=1, "Winnings"=0.0, "Profit"=-120.0}, "Cash Stats"={"Hands Won"=0, "Hands Played"=0, "Hands Dealt"=0, "All-Ins"=0, "Profit"=6.75}}], [{"Player Name"="Andrew", "Date Updated"=timestamp(3698352000 s since 1904-01-01), "Tournament Stats"={"Hands Won"=745, "Hands Played"=2228, "Hands Dealt"=5686, "All-Ins"=169, "Entered"=40, "Winnings"=785.66, "Profit"=-679.15}, "Cash Stats"={"Hands Won"=1691, "Hands Played"=5036, "Hands Dealt"=11645, "All-Ins"=300, "Profit"=-195.0}}, {"Player Name"="Brian", "Date Updated"=timestamp(3698352000 s since 1904-01-01), "Tournament Stats"={"Hands Won"=1049, "Hands Played"=2826, "Hands Dealt"=6323, "All-Ins"=331, "Entered"=53, "Winnings"=1307.11, "Profit"=-47.7}, "Cash Stats"={"Hands Won"=2712, "Hands Played"=7619, "Hands Dealt"=13310, "All-Ins"=444, "Profit"=1902.25}}, {"Player Name"="Daniel", "Date Updated"=timestamp(3698352000 s since 1904-01-01), "Tournament Stats"={"Hands Won"=173, "Hands Played"=476, "Hands Dealt"=1223, "All-Ins"=38, "Entered"=9, "Winnings"=320.0, "Profit"=-20.0}, "Cash Stats"={"Hands Won"=0, "Hands Played"=0, "Hands Dealt"=0, "All-Ins"=0, "Profit"=0.0}}, {"Player Name"="David", "Date Updated"=timestamp(3698352000 s since 1904-01-01), "Tournament Stats"={"Hands Won"=989, "Hands Played"=2209, "Hands Dealt"=5546, "All-Ins"=206, "Entered"=41, "Winnings"=1934.16, "Profit"=574.16}, "Cash Stats"={"Hands Won"=0, "Hands Played"=0, "Hands Dealt"=0, "All-Ins"=0, "Profit"=0.0}}, {"Player Name"="Dennis", "Date Updated"=timestamp(3698352000 s since 1904-01-01), "Tournament Stats"={"Hands Won"=390, "Hands Played"=991, "Hands Dealt"=2790, "All-Ins"=93, "Entered"=20, "Winnings"=1351.83, "Profit"=617.02}, "Cash Stats"={"Hands Won"=79, "Hands Played"=242, "Hands Dealt"=466, "All-Ins"=26, "Profit"=-12.75}}, {"Player Name"="Doug", "Date Updated"=timestamp(3698352000 s since 1904-01-01), "Tournament Stats"={"Hands Won"=191, "Hands Played"=550, "Hands Dealt"=1035, "All-Ins"=61, "Entered"=14, "Winnings"=225.0, "Profit"=-89.81}, "Cash Stats"={"Hands Won"=120, "Hands Played"=285, "Hands Dealt"=428, "All-Ins"=22, "Profit"=-39.5}}, {"Player Name"="Erik", "Date Updated"=timestamp(3698352000 s since 1904-01-01), "Tournament Stats"={"Hands Won"=195, "Hands Played"=696, "Hands Dealt"=2040, "All-Ins"=80, "Entered"=16, "Winnings"=200.66, "Profit"=-259.34}, "Cash Stats"={"Hands Won"=11, "Hands Played"=43, "Hands Dealt"=98, "All-Ins"=7, "Profit"=-34.75}}, {"Player Name"="Ethan", "Date Updated"=timestamp(3698352000 s since 1904-01-01), "Tournament Stats"={"Hands Won"=923, "Hands Played"=2482, "Hands Dealt"=6064, "All-Ins"=247, "Entered"=48, "Winnings"=1270.72, "Profit"=195.91}, "Cash Stats"={"Hands Won"=2681, "Hands Played"=6927, "Hands Dealt"=13273, "All-Ins"=760, "Profit"=1356.0}}, {"Player Name"="Ian", "Date Updated"=timestamp(3698352000 s since 1904-01-01), "Tournament Stats"={"Hands Won"=1727, "Hands Played"=5121, "Hands Dealt"=9854, "All-Ins"=377, "Entered"=77, "Winnings"=1957.52, "Profit"=-407.29}, "Cash Stats"={"Hands Won"=256, "Hands Played"=856, "Hands Dealt"=1326, "All-Ins"=27, "Profit"=-112.0}}, {"Player Name"="Ira", "Date Updated"=timestamp(3698352000 s since 1904-01-01), "Tournament Stats"={"Hands Won"=1563, "Hands Played"=3891, "Hands Dealt"=9600, "All-Ins"=380, "Entered"=80, "Winnings"=2796.14, "Profit"=491.33}, "Cash Stats"={"Hands Won"=1, "Hands Played"=3, "Hands Dealt"=6, "All-Ins"=1, "Profit"=-20.0}}, {"Player Name"="Jason", "Date Updated"=timestamp(3698352000 s since 1904-01-01), "Tournament Stats"={"Hands Won"=137, "Hands Played"=440, "Hands Dealt"=846, "All-Ins"=37, "Entered"=10, "Winnings"=56.0, "Profit"=-324.0}, "Cash Stats"={"Hands Won"=87, "Hands Played"=305, "Hands Dealt"=448, "All-Ins"=19, "Profit"=-77.75}}, {"Player Name"="Jeff", "Date Updated"=timestamp(3698352000 s since 1904-01-01), "Tournament Stats"={"Hands Won"=480, "Hands Played"=1783, "Hands Dealt"=3448, "All-Ins"=111, "Entered"=35, "Winnings"=420.0, "Profit"=-584.81}, "Cash Stats"={"Hands Won"=0, "Hands Played"=0, "Hands Dealt"=0, "All-Ins"=0, "Profit"=0.0}}, {"Player Name"="Jeff-R", "Date Updated"=timestamp(3698352000 s since 1904-01-01), "Tournament Stats"={"Hands Won"=163, "Hands Played"=398, "Hands Dealt"=1069, "All-Ins"=48, "Entered"=9, "Winnings"=256.66, "Profit"=-3.34}, "Cash Stats"={"Hands Won"=10, "Hands Played"=25, "Hands Dealt"=60, "All-Ins"=3, "Profit"=-40.0}}, {"Player Name"="Joe", "Date Updated"=timestamp(3698352000 s since 1904-01-01), "Tournament Stats"={"Hands Won"=7, "Hands Played"=25, "Hands Dealt"=96, "All-Ins"=4, "Entered"=1, "Winnings"=0.0, "Profit"=-60.0}, "Cash Stats"={"Hands Won"=40, "Hands Played"=136, "Hands Dealt"=192, "All-Ins"=13, "Profit"=-132.5}}, {"Player Name"="Joe-Hockman", "Date Updated"=timestamp(3698352000 s since 1904-01-01), "Tournament Stats"={"Hands Won"=3, "Hands Played"=26, "Hands Dealt"=56, "All-Ins"=2, "Entered"=1, "Winnings"=0.0, "Profit"=-40.0}, "Cash Stats"={"Hands Won"=0, "Hands Played"=0, "Hands Dealt"=0, "All-Ins"=0, "Profit"=0.0}}, {"Player Name"="Jonathan-H", "Date Updated"=timestamp(3698352000 s since 1904-01-01), "Tournament Stats"={"Hands Won"=1456, "Hands Played"=3067, "Hands Dealt"=9895, "All-Ins"=424, "Entered"=78, "Winnings"=3077.49, "Profit"=762.68}, "Cash Stats"={"Hands Won"=2527, "Hands Played"=6487, "Hands Dealt"=11380, "All-Ins"=504, "Profit"=1226.5}}, {"Player Name"="Jonathan-M", "Date Updated"=timestamp(3698352000 s since 1904-01-01), "Tournament Stats"={"Hands Won"=2303, "Hands Played"=4639, "Hands Dealt"=10158, "All-Ins"=695, "Entered"=80, "Winnings"=3723.66, "Profit"=1128.85}, "Cash Stats"={"Hands Won"=6370, "Hands Played"=12258, "Hands Dealt"=16919, "All-Ins"=1450, "Profit"=-4255.25}}, {"Player Name"="Mark", "Date Updated"=timestamp(3698352000 s since 1904-01-01), "Tournament Stats"={"Hands Won"=1220, "Hands Played"=2434, "Hands Dealt"=7003, "All-Ins"=323, "Entered"=49, "Winnings"=3075.83, "Profit"=1615.83}, "Cash Stats"={"Hands Won"=984, "Hands Played"=2323, "Hands Dealt"=5269, "All-Ins"=110, "Profit"=895.25}}, {"Player Name"="Marty", "Date Updated"=timestamp(3698352000 s since 1904-01-01), "Tournament Stats"={"Hands Won"=1533, "Hands Played"=3804, "Hands Dealt"=9931, "All-Ins"=415, "Entered"=71, "Winnings"=2027.99, "Profit"=197.99}, "Cash Stats"={"Hands Won"=242, "Hands Played"=729, "Hands Dealt"=1673, "All-Ins"=41, "Profit"=-120.25}}, {"Player Name"="Matt-H", "Date Updated"=timestamp(3698352000 s since 1904-01-01), "Tournament Stats"={"Hands Won"=54, "Hands Played"=147, "Hands Dealt"=285, "All-Ins"=9, "Entered"=4, "Winnings"=34.0, "Profit"=-66.0}, "Cash Stats"={"Hands Won"=0, "Hands Played"=0, "Hands Dealt"=0, "All-Ins"=0, "Profit"=0.0}}, {"Player Name"="Matt-R", "Date Updated"=timestamp(3698352000 s since 1904-01-01), "Tournament Stats"={"Hands Won"=1162, "Hands Played"=2870, "Hands Dealt"=8286, "All-Ins"=394, "Entered"=58, "Winnings"=1520.16, "Profit"=-274.65}, "Cash Stats"={"Hands Won"=288, "Hands Played"=709, "Hands Dealt"=1660, "All-Ins"=104, "Profit"=-121.0}}, {"Player Name"="MikeDolan", "Date Updated"=timestamp(3698352000 s since 1904-01-01), "Tournament Stats"={"Hands Won"=598, "Hands Played"=1696, "Hands Dealt"=4337, "All-Ins"=198, "Entered"=30, "Winnings"=1025.66, "Profit"=85.66}, "Cash Stats"={"Hands Won"=32, "Hands Played"=117, "Hands Dealt"=225, "All-Ins"=14, "Profit"=-66.0}}, {"Player Name"="Nate", "Date Updated"=timestamp(3698352000 s since 1904-01-01), "Tournament Stats"={"Hands Won"=184, "Hands Played"=494, "Hands Dealt"=1384, "All-Ins"=42, "Entered"=14, "Winnings"=234.0, "Profit"=-36.0}, "Cash Stats"={"Hands Won"=0, "Hands Played"=0, "Hands Dealt"=0, "All-Ins"=0, "Profit"=0.0}}, {"Player Name"="Oren", "Date Updated"=timestamp(3698352000 s since 1904-01-01), "Tournament Stats"={"Hands Won"=919, "Hands Played"=2146, "Hands Dealt"=6083, "All-Ins"=197, "Entered"=52, "Winnings"=1157.32, "Profit"=-497.49}, "Cash Stats"={"Hands Won"=19, "Hands Played"=76, "Hands Dealt"=168, "All-Ins"=10, "Profit"=-140.0}}, {"Player Name"="Tom", "Date Updated"=timestamp(3698352000 s since 1904-01-01), "Tournament Stats"={"Hands Won"=15, "Hands Played"=39, "Hands Dealt"=107, "All-Ins"=3, "Entered"=1, "Winnings"=0.0, "Profit"=-120.0}, "Cash Stats"={"Hands Won"=0, "Hands Played"=0, "Hands Dealt"=0, "All-Ins"=0, "Profit"=6.75}}], [{"Player Name"="Andrew", "Date Updated"=timestamp(3698694000 s since 1904-01-01), "Tournament Stats"={"Hands Won"=752, "Hands Played"=2264, "Hands Dealt"=5813, "All-Ins"=174, "Entered"=42, "Winnings"=785.66, "Profit"=-679.15}, "Cash Stats"={"Hands Won"=1769, "Hands Played"=5256, "Hands Dealt"=12108, "All-Ins"=307, "Profit"=-195.0}}, {"Player Name"="Brian", "Date Updated"=timestamp(3698694000 s since 1904-01-01), "Tournament Stats"={"Hands Won"=1057, "Hands Played"=2847, "Hands Dealt"=6385, "All-Ins"=335, "Entered"=54, "Winnings"=1307.11, "Profit"=-47.7}, "Cash Stats"={"Hands Won"=2760, "Hands Played"=7774, "Hands Dealt"=13600, "All-Ins"=450, "Profit"=1902.25}}, {"Player Name"="Daniel", "Date Updated"=timestamp(3698694000 s since 1904-01-01), "Tournament Stats"={"Hands Won"=188, "Hands Played"=509, "Hands Dealt"=1337, "All-Ins"=44, "Entered"=10, "Winnings"=320.0, "Profit"=-20.0}, "Cash Stats"={"Hands Won"=0, "Hands Played"=0, "Hands Dealt"=0, "All-Ins"=0, "Profit"=0.0}}, {"Player Name"="David", "Date Updated"=timestamp(3698694000 s since 1904-01-01), "Tournament Stats"={"Hands Won"=997, "Hands Played"=2233, "Hands Dealt"=5608, "All-Ins"=208, "Entered"=42, "Winnings"=1934.16, "Profit"=574.16}, "Cash Stats"={"Hands Won"=0, "Hands Played"=0, "Hands Dealt"=0, "All-Ins"=0, "Profit"=0.0}}, {"Player Name"="Dennis", "Date Updated"=timestamp(3698694000 s since 1904-01-01), "Tournament Stats"={"Hands Won"=396, "Hands Played"=1023, "Hands Dealt"=2885, "All-Ins"=95, "Entered"=21, "Winnings"=1351.83, "Profit"=617.02}, "Cash Stats"={"Hands Won"=113, "Hands Played"=327, "Hands Dealt"=656, "All-Ins"=32, "Profit"=-12.75}}, {"Player Name"="Doug", "Date Updated"=timestamp(3698694000 s since 1904-01-01), "Tournament Stats"={"Hands Won"=191, "Hands Played"=550, "Hands Dealt"=1035, "All-Ins"=61, "Entered"=14, "Winnings"=225.0, "Profit"=-89.81}, "Cash Stats"={"Hands Won"=120, "Hands Played"=285, "Hands Dealt"=428, "All-Ins"=22, "Profit"=-39.5}}, {"Player Name"="Erik", "Date Updated"=timestamp(3698694000 s since 1904-01-01), "Tournament Stats"={"Hands Won"=201, "Hands Played"=724, "Hands Dealt"=2110, "All-Ins"=82, "Entered"=17, "Winnings"=200.66, "Profit"=-259.34}, "Cash Stats"={"Hands Won"=11, "Hands Played"=43, "Hands Dealt"=98, "All-Ins"=7, "Profit"=-34.75}}, {"Player Name"="Ethan", "Date Updated"=timestamp(3698694000 s since 1904-01-01), "Tournament Stats"={"Hands Won"=958, "Hands Played"=2547, "Hands Dealt"=6232, "All-Ins"=252, "Entered"=49, "Winnings"=1270.72, "Profit"=195.91}, "Cash Stats"={"Hands Won"=2756, "Hands Played"=7133, "Hands Dealt"=13652, "All-Ins"=785, "Profit"=1356.0}}, {"Player Name"="Ian", "Date Updated"=timestamp(3698694000 s since 1904-01-01), "Tournament Stats"={"Hands Won"=1760, "Hands Played"=5228, "Hands Dealt"=10106, "All-Ins"=389, "Entered"=79, "Winnings"=1957.52, "Profit"=-407.29}, "Cash Stats"={"Hands Won"=261, "Hands Played"=879, "Hands Dealt"=1373, "All-Ins"=30, "Profit"=-112.0}}, {"Player Name"="Ira", "Date Updated"=timestamp(3698694000 s since 1904-01-01), "Tournament Stats"={"Hands Won"=1607, "Hands Played"=3991, "Hands Dealt"=9834, "All-Ins"=392, "Entered"=82, "Winnings"=2796.14, "Profit"=491.33}, "Cash Stats"={"Hands Won"=1, "Hands Played"=3, "Hands Dealt"=6, "All-Ins"=1, "Profit"=-20.0}}, {"Player Name"="Jason", "Date Updated"=timestamp(3698694000 s since 1904-01-01), "Tournament Stats"={"Hands Won"=137, "Hands Played"=440, "Hands Dealt"=846, "All-Ins"=37, "Entered"=10, "Winnings"=56.0, "Profit"=-324.0}, "Cash Stats"={"Hands Won"=87, "Hands Played"=305, "Hands Dealt"=448, "All-Ins"=19, "Profit"=-77.75}}, {"Player Name"="Jeff", "Date Updated"=timestamp(3698694000 s since 1904-01-01), "Tournament Stats"={"Hands Won"=480, "Hands Played"=1783, "Hands Dealt"=3448, "All-Ins"=111, "Entered"=35, "Winnings"=420.0, "Profit"=-584.81}, "Cash Stats"={"Hands Won"=0, "Hands Played"=0, "Hands Dealt"=0, "All-Ins"=0, "Profit"=0.0}}, {"Player Name"="Jeff-R", "Date Updated"=timestamp(3698694000 s since 1904-01-01), "Tournament Stats"={"Hands Won"=163, "Hands Played"=398, "Hands Dealt"=1069, "All-Ins"=48, "Entered"=9, "Winnings"=256.66, "Profit"=-3.34}, "Cash Stats"={"Hands Won"=10, "Hands Played"=25, "Hands Dealt"=60, "All-Ins"=3, "Profit"=-40.0}}, {"Player Name"="Joe", "Date Updated"=timestamp(3698694000 s since 1904-01-01), "Tournament Stats"={"Hands Won"=7, "Hands Played"=25, "Hands Dealt"=96, "All-Ins"=4, "Entered"=1, "Winnings"=0.0, "Profit"=-60.0}, "Cash Stats"={"Hands Won"=40, "Hands Played"=136, "Hands Dealt"=192, "All-Ins"=13, "Profit"=-132.5}}, {"Player Name"="Joe-Hockman", "Date Updated"=timestamp(3698694000 s since 1904-01-01), "Tournament Stats"={"Hands Won"=3, "Hands Played"=26, "Hands Dealt"=56, "All-Ins"=2, "Entered"=1, "Winnings"=0.0, "Profit"=-40.0}, "Cash Stats"={"Hands Won"=0, "Hands Played"=0, "Hands Dealt"=0, "All-Ins"=0, "Profit"=0.0}}, {"Player Name"="Jonathan-H", "Date Updated"=timestamp(3698694000 s since 1904-01-01), "Tournament Stats"={"Hands Won"=1504, "Hands Played"=3156, "Hands Dealt"=10127, "All-Ins"=432, "Entered"=80, "Winnings"=3077.49, "Profit"=762.68}, "Cash Stats"={"Hands Won"=2596, "Hands Played"=6631, "Hands Dealt"=11599, "All-Ins"=515, "Profit"=1226.5}}, {"Player Name"="Jonathan-M", "Date Updated"=timestamp(3698694000 s since 1904-01-01), "Tournament Stats"={"Hands Won"=2370, "Hands Played"=4740, "Hands Dealt"=10373, "All-Ins"=703, "Entered"=82, "Winnings"=3723.66, "Profit"=1128.85}, "Cash Stats"={"Hands Won"=6460, "Hands Played"=12437, "Hands Dealt"=17138, "All-Ins"=1466, "Profit"=-4255.25}}, {"Player Name"="Mark", "Date Updated"=timestamp(3698694000 s since 1904-01-01), "Tournament Stats"={"Hands Won"=1253, "Hands Played"=2501, "Hands Dealt"=7183, "All-Ins"=335, "Entered"=51, "Winnings"=3075.83, "Profit"=1615.83}, "Cash Stats"={"Hands Won"=1029, "Hands Played"=2446, "Hands Dealt"=5657, "All-Ins"=123, "Profit"=895.25}}, {"Player Name"="Marty", "Date Updated"=timestamp(3698694000 s since 1904-01-01), "Tournament Stats"={"Hands Won"=1575, "Hands Played"=3904, "Hands Dealt"=10212, "All-Ins"=418, "Entered"=73, "Winnings"=2027.99, "Profit"=197.99}, "Cash Stats"={"Hands Won"=249, "Hands Played"=754, "Hands Dealt"=1728, "All-Ins"=42, "Profit"=-120.25}}, {"Player Name"="Matt-H", "Date Updated"=timestamp(3698694000 s since 1904-01-01), "Tournament Stats"={"Hands Won"=54, "Hands Played"=147, "Hands Dealt"=285, "All-Ins"=9, "Entered"=4, "Winnings"=34.0, "Profit"=-66.0}, "Cash Stats"={"Hands Won"=0, "Hands Played"=0, "Hands Dealt"=0, "All-Ins"=0, "Profit"=0.0}}, {"Player Name"="Matt-R", "Date Updated"=timestamp(3698694000 s since 1904-01-01), "Tournament Stats"={"Hands Won"=1206, "Hands Played"=2992, "Hands Dealt"=8581, "All-Ins"=406, "Entered"=60, "Winnings"=1520.16, "Profit"=-274.65}, "Cash Stats"={"Hands Won"=296, "Hands Played"=734, "Hands Dealt"=1722, "All-Ins"=111, "Profit"=-121.0}}, {"Player Name"="MikeDolan", "Date Updated"=timestamp(3698694000 s since 1904-01-01), "Tournament Stats"={"Hands Won"=602, "Hands Played"=1709, "Hands Dealt"=4358, "All-Ins"=200, "Entered"=31, "Winnings"=1025.66, "Profit"=85.66}, "Cash Stats"={"Hands Won"=32, "Hands Played"=117, "Hands Dealt"=225, "All-Ins"=14, "Profit"=-66.0}}, {"Player Name"="Nate", "Date Updated"=timestamp(3698694000 s since 1904-01-01), "Tournament Stats"={"Hands Won"=184, "Hands Played"=494, "Hands Dealt"=1384, "All-Ins"=42, "Entered"=14, "Winnings"=234.0, "Profit"=-36.0}, "Cash Stats"={"Hands Won"=0, "Hands Played"=0, "Hands Dealt"=0, "All-Ins"=0, "Profit"=0.0}}, {"Player Name"="Oren", "Date Updated"=timestamp(3698694000 s since 1904-01-01), "Tournament Stats"={"Hands Won"=948, "Hands Played"=2205, "Hands Dealt"=6244, "All-Ins"=199, "Entered"=53, "Winnings"=1157.32, "Profit"=-497.49}, "Cash Stats"={"Hands Won"=19, "Hands Played"=76, "Hands Dealt"=168, "All-Ins"=10, "Profit"=-140.0}}, {"Player Name"="Tom", "Date Updated"=timestamp(3698694000 s since 1904-01-01), "Tournament Stats"={"Hands Won"=28, "Hands Played"=87, "Hands Dealt"=200, "All-Ins"=7, "Entered"=2, "Winnings"=0.0, "Profit"=-120.0}, "Cash Stats"={"Hands Won"=11, "Hands Played"=35, "Hands Dealt"=60, "All-Ins"=2, "Profit"=6.75}}], [{"Player Name"="Andrew", "Date Updated"=timestamp(3699298800 s since 1904-01-01), "Tournament Stats"={"Hands Won"=757, "Hands Played"=2299, "Hands Dealt"=5915, "All-Ins"=179, "Entered"=43, "Winnings"=785.66, "Profit"=-679.15}, "Cash Stats"={"Hands Won"=1830, "Hands Played"=5456, "Hands Dealt"=12562, "All-Ins"=316, "Profit"=-195.0}}, {"Player Name"="Brian", "Date Updated"=timestamp(3699298800 s since 1904-01-01), "Tournament Stats"={"Hands Won"=1067, "Hands Played"=2883, "Hands Dealt"=6486, "All-Ins"=337, "Entered"=55, "Winnings"=1307.11, "Profit"=-47.7}, "Cash Stats"={"Hands Won"=2853, "Hands Played"=8063, "Hands Dealt"=14064, "All-Ins"=465, "Profit"=1902.25}}, {"Player Name"="Daniel", "Date Updated"=timestamp(3699298800 s since 1904-01-01), "Tournament Stats"={"Hands Won"=207, "Hands Played"=555, "Hands Dealt"=1509, "All-Ins"=46, "Entered"=11, "Winnings"=320.0, "Profit"=-20.0}, "Cash Stats"={"Hands Won"=0, "Hands Played"=0, "Hands Dealt"=0, "All-Ins"=0, "Profit"=0.0}}, {"Player Name"="David", "Date Updated"=timestamp(3699298800 s since 1904-01-01), "Tournament Stats"={"Hands Won"=1008, "Hands Played"=2261, "Hands Dealt"=5690, "All-Ins"=212, "Entered"=43, "Winnings"=1934.16, "Profit"=574.16}, "Cash Stats"={"Hands Won"=0, "Hands Played"=0, "Hands Dealt"=0, "All-Ins"=0, "Profit"=0.0}}, {"Player Name"="Dennis", "Date Updated"=timestamp(3699298800 s since 1904-01-01), "Tournament Stats"={"Hands Won"=445, "Hands Played"=1136, "Hands Dealt"=3195, "All-Ins"=102, "Entered"=23, "Winnings"=1351.83, "Profit"=617.02}, "Cash Stats"={"Hands Won"=114, "Hands Played"=332, "Hands Dealt"=672, "All-Ins"=34, "Profit"=-12.75}}, {"Player Name"="Doug", "Date Updated"=timestamp(3699298800 s since 1904-01-01), "Tournament Stats"={"Hands Won"=191, "Hands Played"=550, "Hands Dealt"=1035, "All-Ins"=61, "Entered"=14, "Winnings"=225.0, "Profit"=-89.81}, "Cash Stats"={"Hands Won"=120, "Hands Played"=285, "Hands Dealt"=428, "All-Ins"=22, "Profit"=-39.5}}, {"Player Name"="Erik", "Date Updated"=timestamp(3699298800 s since 1904-01-01), "Tournament Stats"={"Hands Won"=201, "Hands Played"=724, "Hands Dealt"=2110, "All-Ins"=82, "Entered"=17, "Winnings"=200.66, "Profit"=-259.34}, "Cash Stats"={"Hands Won"=11, "Hands Played"=43, "Hands Dealt"=98, "All-Ins"=7, "Profit"=-34.75}}, {"Player Name"="Ethan", "Date Updated"=timestamp(3699298800 s since 1904-01-01), "Tournament Stats"={"Hands Won"=985, "Hands Played"=2603, "Hands Dealt"=6375, "All-Ins"=257, "Entered"=50, "Winnings"=1270.72, "Profit"=195.91}, "Cash Stats"={"Hands Won"=2872, "Hands Played"=7450, "Hands Dealt"=14199, "All-Ins"=811, "Profit"=1356.0}}, {"Player Name"="Ian", "Date Updated"=timestamp(3699298800 s since 1904-01-01), "Tournament Stats"={"Hands Won"=1801, "Hands Played"=5359, "Hands Dealt"=10407, "All-Ins"=395, "Entered"=81, "Winnings"=1957.52, "Profit"=-407.29}, "Cash Stats"={"Hands Won"=271, "Hands Played"=925, "Hands Dealt"=1468, "All-Ins"=33, "Profit"=-112.0}}, {"Player Name"="Ira", "Date Updated"=timestamp(3699298800 s since 1904-01-01), "Tournament Stats"={"Hands Won"=1648, "Hands Played"=4095, "Hands Dealt"=10027, "All-Ins"=398, "Entered"=84, "Winnings"=2796.14, "Profit"=491.33}, "Cash Stats"={"Hands Won"=1, "Hands Played"=3, "Hands Dealt"=6, "All-Ins"=1, "Profit"=-20.0}}, {"Player Name"="Jason", "Date Updated"=timestamp(3699298800 s since 1904-01-01), "Tournament Stats"={"Hands Won"=162, "Hands Played"=520, "Hands Dealt"=981, "All-Ins"=39, "Entered"=11, "Winnings"=56.0, "Profit"=-324.0}, "Cash Stats"={"Hands Won"=87, "Hands Played"=305, "Hands Dealt"=448, "All-Ins"=19, "Profit"=-77.75}}, {"Player Name"="Jeff", "Date Updated"=timestamp(3699298800 s since 1904-01-01), "Tournament Stats"={"Hands Won"=481, "Hands Played"=1805, "Hands Dealt"=3494, "All-Ins"=113, "Entered"=36, "Winnings"=420.0, "Profit"=-584.81}, "Cash Stats"={"Hands Won"=0, "Hands Played"=0, "Hands Dealt"=0, "All-Ins"=0, "Profit"=0.0}}, {"Player Name"="Jeff-R", "Date Updated"=timestamp(3699298800 s since 1904-01-01), "Tournament Stats"={"Hands Won"=163, "Hands Played"=398, "Hands Dealt"=1069, "All-Ins"=48, "Entered"=9, "Winnings"=256.66, "Profit"=-3.34}, "Cash Stats"={"Hands Won"=10, "Hands Played"=25, "Hands Dealt"=60, "All-Ins"=3, "Profit"=-40.0}}, {"Player Name"="Joe", "Date Updated"=timestamp(3699298800 s since 1904-01-01), "Tournament Stats"={"Hands Won"=7, "Hands Played"=25, "Hands Dealt"=96, "All-Ins"=4, "Entered"=1, "Winnings"=0.0, "Profit"=-60.0}, "Cash Stats"={"Hands Won"=59, "Hands Played"=197, "Hands Dealt"=315, "All-Ins"=25, "Profit"=-132.5}}, {"Player Name"="Joe-Hockman", "Date Updated"=timestamp(3699298800 s since 1904-01-01), "Tournament Stats"={"Hands Won"=3, "Hands Played"=26, "Hands Dealt"=56, "All-Ins"=2, "Entered"=1, "Winnings"=0.0, "Profit"=-40.0}, "Cash Stats"={"Hands Won"=0, "Hands Played"=0, "Hands Dealt"=0, "All-Ins"=0, "Profit"=0.0}}, {"Player Name"="Jonathan-H", "Date Updated"=timestamp(3699298800 s since 1904-01-01), "Tournament Stats"={"Hands Won"=1509, "Hands Played"=3177, "Hands Dealt"=10200, "All-Ins"=438, "Entered"=82, "Winnings"=3077.49, "Profit"=762.68}, "Cash Stats"={"Hands Won"=2627, "Hands Played"=6717, "Hands Dealt"=11746, "All-Ins"=517, "Profit"=1226.5}}, {"Player Name"="Jonathan-M", "Date Updated"=timestamp(3699298800 s since 1904-01-01), "Tournament Stats"={"Hands Won"=2375, "Hands Played"=4763, "Hands Dealt"=10427, "All-Ins"=710, "Entered"=84, "Winnings"=3723.66, "Profit"=1128.85}, "Cash Stats"={"Hands Won"=6742, "Hands Played"=12974, "Hands Dealt"=17902, "All-Ins"=1505, "Profit"=-4255.25}}, {"Player Name"="Mark", "Date Updated"=timestamp(3699298800 s since 1904-01-01), "Tournament Stats"={"Hands Won"=1300, "Hands Played"=2585, "Hands Dealt"=7494, "All-Ins"=341, "Entered"=53, "Winnings"=3075.83, "Profit"=1615.83}, "Cash Stats"={"Hands Won"=1120, "Hands Played"=2693, "Hands Dealt"=6292, "All-Ins"=139, "Profit"=895.25}}, {"Player Name"="Marty", "Date Updated"=timestamp(3699298800 s since 1904-01-01), "Tournament Stats"={"Hands Won"=1601, "Hands Played"=3973, "Hands Dealt"=10396, "All-Ins"=426, "Entered"=75, "Winnings"=2027.99, "Profit"=197.99}, "Cash Stats"={"Hands Won"=297, "Hands Played"=870, "Hands Dealt"=1961, "All-Ins"=43, "Profit"=-120.25}}, {"Player Name"="Matt-H", "Date Updated"=timestamp(3699298800 s since 1904-01-01), "Tournament Stats"={"Hands Won"=54, "Hands Played"=147, "Hands Dealt"=285, "All-Ins"=9, "Entered"=4, "Winnings"=34.0, "Profit"=-66.0}, "Cash Stats"={"Hands Won"=0, "Hands Played"=0, "Hands Dealt"=0, "All-Ins"=0, "Profit"=0.0}}, {"Player Name"="Matt-R", "Date Updated"=timestamp(3699298800 s since 1904-01-01), "Tournament Stats"={"Hands Won"=1255, "Hands Played"=3119, "Hands Dealt"=8912, "All-Ins"=422, "Entered"=62, "Winnings"=1520.16, "Profit"=-274.65}, "Cash Stats"={"Hands Won"=303, "Hands Played"=754, "Hands Dealt"=1762, "All-Ins"=113, "Profit"=-121.0}}, {"Player Name"="MikeDolan", "Date Updated"=timestamp(3699298800 s since 1904-01-01), "Tournament Stats"={"Hands Won"=615, "Hands Played"=1748, "Hands Dealt"=4469, "All-Ins"=206, "Entered"=32, "Winnings"=1025.66, "Profit"=85.66}, "Cash Stats"={"Hands Won"=32, "Hands Played"=117, "Hands Dealt"=225, "All-Ins"=14, "Profit"=-66.0}}, {"Player Name"="Nate", "Date Updated"=timestamp(3699298800 s since 1904-01-01), "Tournament Stats"={"Hands Won"=184, "Hands Played"=494, "Hands Dealt"=1384, "All-Ins"=42, "Entered"=14, "Winnings"=234.0, "Profit"=-36.0}, "Cash Stats"={"Hands Won"=0, "Hands Played"=0, "Hands Dealt"=0, "All-Ins"=0, "Profit"=0.0}}, {"Player Name"="Oren", "Date Updated"=timestamp(3699298800 s since 1904-01-01), "Tournament Stats"={"Hands Won"=964, "Hands Played"=2253, "Hands Dealt"=6361, "All-Ins"=204, "Entered"=54, "Winnings"=1157.32, "Profit"=-497.49}, "Cash Stats"={"Hands Won"=19, "Hands Played"=76, "Hands Dealt"=168, "All-Ins"=10, "Profit"=-140.0}}, {"Player Name"="Tom", "Date Updated"=timestamp(3699298800 s since 1904-01-01), "Tournament Stats"={"Hands Won"=61, "Hands Played"=160, "Hands Dealt"=357, "All-Ins"=11, "Entered"=3, "Winnings"=0.0, "Profit"=-120.0}, "Cash Stats"={"Hands Won"=39, "Hands Played"=117, "Hands Dealt"=202, "All-Ins"=7, "Profit"=6.75}}]] {"Date Updated" format="%<%m/%d/%Y>T"}
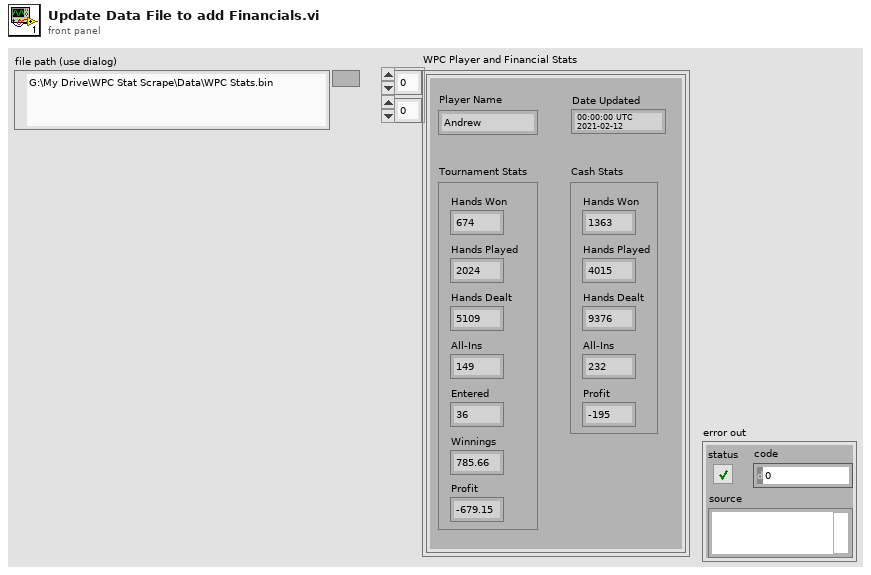
[diagram p1: front panel]
types:
  T1 = typedef "WPC Player and Financial Stats.ctl" = cluster{"Player Name":string, "Date Updated":timestamp, "Tournament Stats":cluster{"Hands Won":u32, "Hands Played":u32, "Hands Dealt":u32, "All-Ins":u32, "Entered":u32, "Winnings":dbl, "Profit":dbl}, "Cash Stats":cluster{"Hands Won":u32, "Hands Played":u32, "Hands Dealt":u32, "All-Ins":u32, "Profit":dbl}}
  T2 = enum16{"open", "replace", "create", "open or create", "replace or create", "replace or create with confirmation"}
  T3 = cluster{"Player Name":string, "Date Updated":timestamp, "Tournament Stats":cluster{"Hands Won":dbl, "Hands Played":dbl, "Hands Dealt":dbl, "All-Ins":dbl, "Entered":dbl}, "Cash Stats":cluster{"Hands Won":dbl, "Hands Played":dbl, "Hands Dealt":dbl, "All-Ins":dbl}}[][]
  T4 = cluster{"Player":string, "Tournament Winings":dbl, "Tournament Profit":dbl}[]
  T5 = cluster{"Hands Won":dbl, "Hands Played":dbl, "Hands Dealt":dbl, "All-Ins":dbl, "Entered":dbl}
  T6 = cluster{"Hands Won":dbl, "Hands Played":dbl, "Hands Dealt":dbl, "All-Ins":dbl}
  T7 = cluster{"Player":string, "Tournament Winings":dbl, "Tournament Profit":dbl}
  T8 = cluster{"[0]":dbl, "[1]":dbl, "[2]":dbl, "[3]":dbl, "[4]":dbl, "[5]":dbl, "[6]":dbl}
  T9 = cluster{"[0]":dbl, "[1]":dbl, "[2]":dbl, "[3]":dbl, "[4]":dbl}
  T10 = cluster{"Player Name":string, "Date Updated":timestamp, cluster{"[0]":dbl, "[1]":dbl, "[2]":dbl, "[3]":dbl, "[4]":dbl, "[5]":dbl, "[6]":dbl}, cluster{"[0]":dbl, "[1]":dbl, "[2]":dbl, "[3]":dbl, "[4]":dbl}}
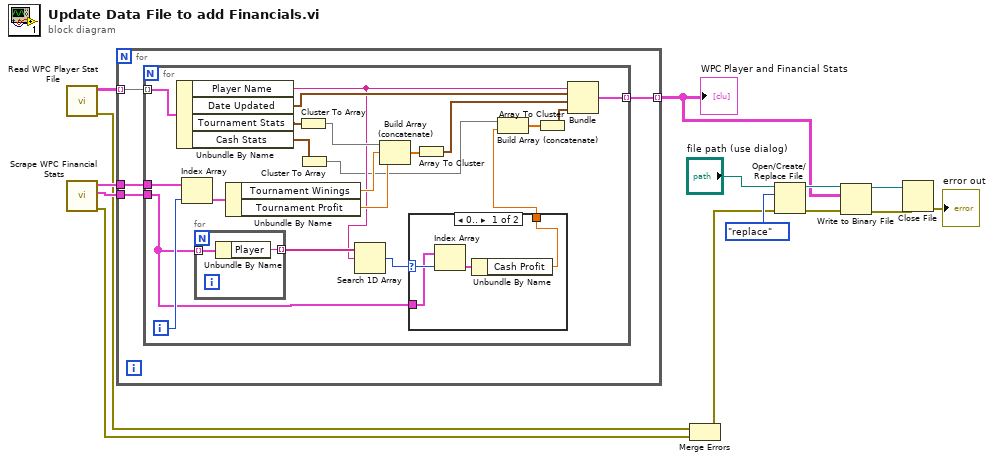
[diagram p0: block diagram]
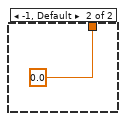
[diagram p2: hidden frame]
diagram:
  n1 = call "Read WPC Player Stat File.vi"() -> ("error out"=w5:errorcluster, "Full WPC Player Stats"=w14:T3)  [unwired: 9 in, 1 out]
  n2 = call "Scrape WPC Financial Stats.vi"() -> ("error out"=w4:errorcluster, "WPC Financial Cash Stats"=w12:cluster{"Player":string, "Cash Profit":dbl}[], "WPC Financial Tournament Stats"=w13:T4)  [unwired: 9 in]
  n3 = for {
    tunnel: w14 -> [w18] mode=indexing
    tunnel: w13 -> [w17]
    tunnel: w12 -> [w16]
    tunnel: [w15] -> w6 mode=indexing
    n4 = for {
      tunnel: w18 -> [w39] mode=indexing
      tunnel: w17 -> [w38]
      tunnel: w16 -> [w20]
      tunnel: [w19] -> w15 mode=indexing
      i -> [w37]
      n5 = Unbundle By Name(w39) -> ("Player Name"=w27:string, "Date Updated"=w35:timestamp, "Tournament Stats"=w34:T5, "Cash Stats"=w25:T6)
      n6 = Index Array(array=w38, index=w37) -> (element=w36:T7)
      n7 = for {
        tunnel: w20 -> [w46] mode=indexing
        tunnel: [w45] -> w28 mode=indexing
        n8 = Unbundle By Name(w46) -> ("Player"=w45:string)
      }
      n9 = Unbundle By Name(w36) -> ("Tournament Winings"=w32:dbl, "Tournament Profit"=w31:dbl)
      n10 = Cluster To Array(cluster=w34) -> (array=w33:dbl[])
      n11 = Cluster To Array(cluster=w25) -> (array=w24:dbl[])
      n12 = Search 1D Array(1D array=w28, element=w27) -> (index of element=w26:i32)  [unwired: 1 in]
      n13 = Build Array (concatenate)(w33, w32, w31) -> (w30:dbl[])
      n14 = case shown="0.." w26 {
        selector: w26 -> [w43 _]
        tunnel: [w40 0.0] -> w21
        tunnel: w20 -> [w42 _]
        frame 0.. {
          n15 = Index Array(array=w42, index=w43) -> (element=w41:cluster{"Player":string, "Cash Profit":dbl})
          n16 = Unbundle By Name(w41) -> ("Cash Profit"=w40:dbl)
        }
        frame -1, Default {
        }
      }
      n17 = Array To Cluster(array=w30) -> (cluster=w29:T8)
      n18 = Build Array (concatenate)(w24, w21) -> (w23:dbl[])
      n19 = Array To Cluster(array=w23) -> (cluster=w22:T9)
      n20 = Bundle("Player Name"=w27, "Date Updated"=w35, w29, w22) -> (w19:T10)  [unwired: 1 in]
    }
  }
  "WPC Player and Financial Stats" <- w6
  n21 = Merge Errors(w5, w4) -> (w3:errorcluster)
  n22 = Open/Create/Replace File(file path (use dialog)="file path (use dialog)", error in=w3, operation (0:open)=T2."replace") -> (refnum out=w9:refnum<file>, error out=w10:errorcluster)  [unwired: 3 in, 1 out]
  n23 = Write to Binary File(file (use dialog)=w9, data=w6, error in=w10) -> (refnum out=w8:refnum<file>, error out=w7:errorcluster)  [unwired: 3 in, 1 out]
  n24 = Close File(refnum=w8, error in=w7) -> (error out=→"error out":errorcluster)  [unwired: 1 out]
